vi "speed to disc.vi"(0 "task in digital":i32, 1 "data":u8[](array[numeric]), 2 "speed change":dbl format="%#_13g", 3 "change limit":dbl, 4 "speed max limit":dbl format="%#_13g", 5 "speed min limit":dbl format="%#_13g", 6 "speed in":dbl format="%#_13g", 7 "wait time":u32, 8 "task inAnalog":i32, 11 "error in (no error)":errorcluster) -> (21 "task out":i32, 22 "inc":bool, 23 "dec":bool, 24 "no change":bool, 25 "error out":errorcluster)   [LabVIEW 2019]
uses:
  <userlib>/DAQNavi Polymorphic VI/write/DAQNavi Write (Analog DBL 1Chan 1Samp).vi
  <userlib>/DAQNavi Polymorphic VI/write/DAQNavi Write (Digtial 1D U8 NChan 1Samp).vi
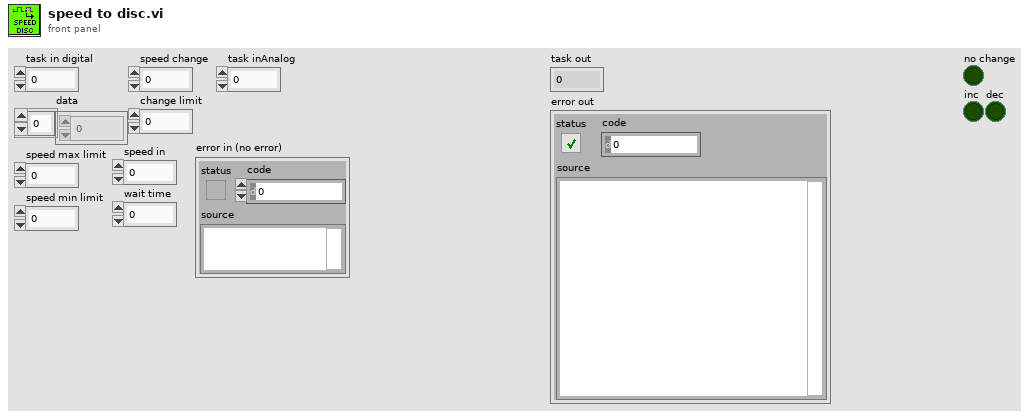
[diagram p1: front panel]
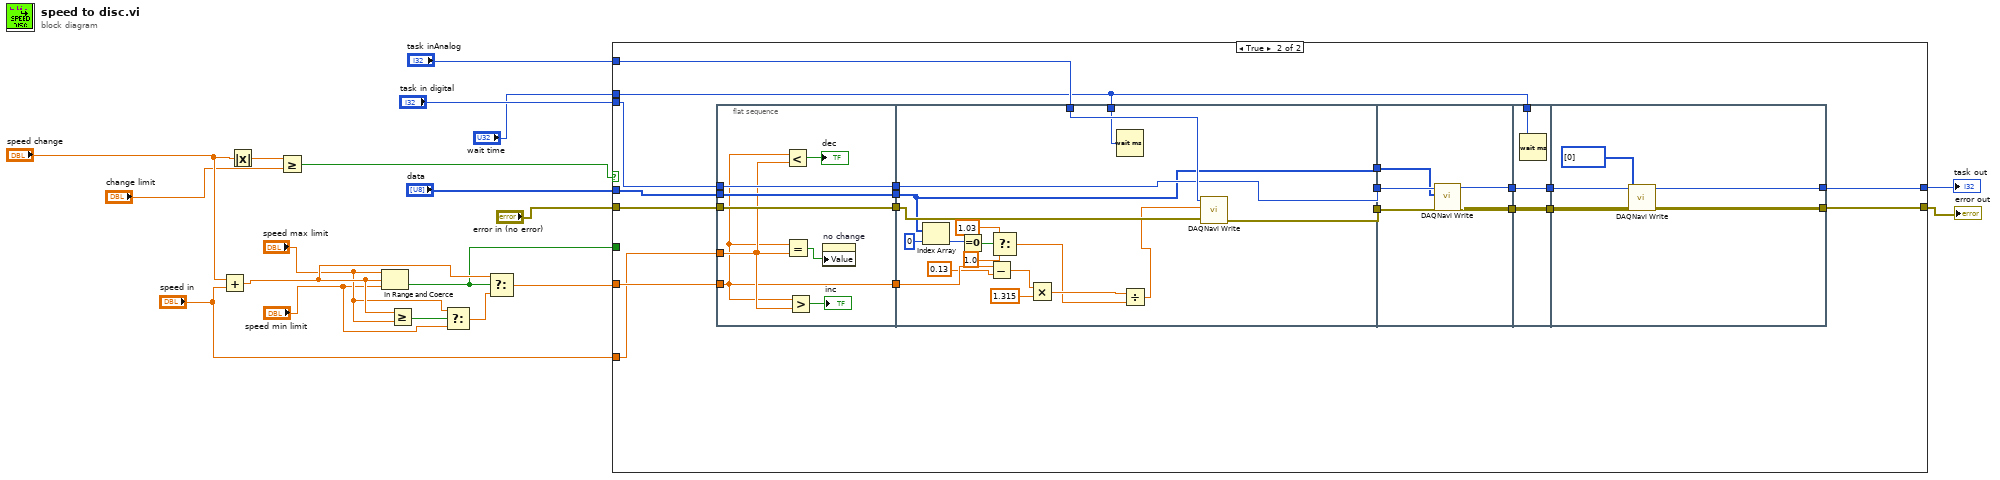
[diagram p0: block diagram]
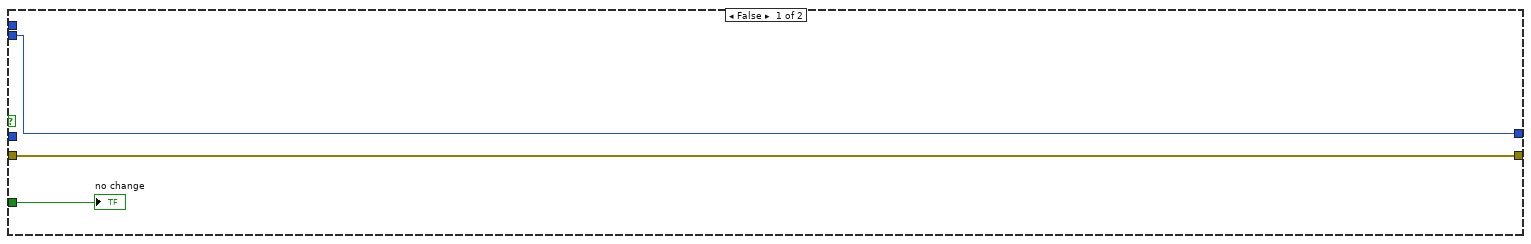
[diagram p2: hidden frame]
diagram:
  n1 = Add(x="speed change", y="speed in") -> (x+y=w17:dbl)
  n2 = Absolute Value(x="speed change") -> (abs(x)=w11:dbl)
  n3 = Greater Or Equal?(x=w11, y="change limit") -> (x >= y?=w8:bool)
  n4 = In Range and Coerce(upper limit="speed max limit", x=w17, lower limit="speed min limit") -> (In Range?=w4:bool)  [unwired: 1 out]
  n5 = Greater Or Equal?(x=w17, y="speed max limit") -> (x >= y?=w16:bool)
  n6 = Select(t="speed max limit", s=w16, f="speed min limit") -> (s? t:f=w13:dbl)
  n7 = Select(t=w17, s=w4, f=w13) -> (s? t:f=w1:dbl)
  n8 = case shown="True" w8 {
    tunnel: "task in digital" -> [w22 w42]
    tunnel: "data" -> [_ w41]
    tunnel: "wait time" -> [_ w23]
    tunnel: w1 -> [_ w37]
    tunnel: "error in (no error)" -> [w21 w40]
    tunnel: [w22 w39] -> w6
    tunnel: [w21 w38] -> w5
    tunnel: w4 -> [w20 _]
    tunnel: "speed in" -> [_ w32]
    tunnel: "task inAnalog" -> [_ w31]
    frame False {
      "no change" <- w20
    }
    frame True {
      n9 = flat-sequence {
        tunnel: w40 -> [w48]
        tunnel: w37 -> [w43]
        tunnel: w41 -> [w49]
        tunnel: w42 -> [w50]
        tunnel: [w50] -> w36
        tunnel: [w49] -> w35
        tunnel: [w43] -> w34
        tunnel: [w48] -> w33
        tunnel: w32 -> [w44]
        tunnel: [w64] -> w30
        tunnel: [w68] -> w29
        tunnel: w31 -> [w67]
        tunnel: w33 -> [w65]
        tunnel: w34 -> [w62]
        tunnel: w35 -> [w60]
        tunnel: w36 -> [w64]
        tunnel: [w60] -> w28
        tunnel: w23 -> [w63]
        tunnel: w30 -> [w71]
        tunnel: [w70] -> w27
        tunnel: w29 -> [w72]
        tunnel: [w72] -> w25
        tunnel: w28 -> [w69]
        tunnel: w27 -> [w75]
        tunnel: [w75] -> w26
        tunnel: w25 -> [w74]
        tunnel: [w74] -> w24
        tunnel: w23 -> [w73]
        tunnel: [w80] -> w39
        tunnel: [w79] -> w38
        tunnel: w24 -> [w76]
        tunnel: w26 -> [w78]
        frame #0 {
          n10 = Less?(x=w43, y=w44) -> (x < y?=→"dec":bool)
          n11 = Equal?(x=w43, y=w44) -> (x = y?=w47:bool)
          n12 = Greater?(x=w43, y=w44) -> (0:→"inc":bool)
          n13 = property on="no change" class="Bool (strict)"("Value"=w47) -> ()  [unwired: 2 in, 2 out]
        }
        frame #1 {
          n14 = Index Array(array=w60, index=0) -> (element=w58:u8)
          n15 = Equal To 0?(x=w58) -> (x = 0?=w57:bool)
          n16 = Subtract(x=w62, y=0.13) -> (x-y=w61:dbl)
          n17 = Select(t=1.03, s=w57, f=1.0) -> (s? t:f=w52:dbl)
          n18 = Multiply(x=w61, y=1.315) -> (x*y=w53:dbl)
          n19 = Wait (ms)(milliseconds to wait=w63) -> ()  [unwired: 1 out]
          n20 = Divide(x=w53, y=w52) -> (x/y=w51:dbl)
          n21 = call-poly <userlib>:"DAQNavi Write.vi"("error in (no error)"=w65, "data"=w51, "task in"=w67) -> ("error out"=w68:errorcluster)  [unwired: 6 in, 2 out]
        }
        frame #2 {
          n22 = call-poly <userlib>:"DAQNavi Write.vi"("data"=w69, "task in"=w71) -> ("task out"=w70:i32)  [unwired: 7 in, 2 out]
        }
        frame #3 {
          n23 = Wait (ms)(milliseconds to wait=w73) -> ()  [unwired: 1 out]
        }
        frame #4 {
          n24 = call-poly <userlib>:"DAQNavi Write.vi"("error in (no error)"=w76, "data"=u8[] [0], "task in"=w78) -> ("error out"=w79:errorcluster, "task out"=w80:i32)  [unwired: 6 in, 1 out]
        }
      }
    }
  }
  "task out" <- w6
  "error out" <- w5
